vi "Run.vi"(8 "error in (no error)":errorcluster caption="entrée d'erreur (pas d'erreur)", 9 "labels_pred":string[][](array[string]), 10 "labels_true":string[][](array[string]), 11 "Contingency_Matrix.lvclass":refnum<class "Contingency_Matrix.lvclass">) -> (0 "error out":errorcluster caption="sortie d'erreur", 2 "Data":T1, 3 "Contingency_Matrix.lvclass":refnum<class "Contingency_Matrix.lvclass">)   [LabVIEW 2020, in "Contingency_Matrix.lvclass"]
doc: "Returns :\n\n- contingency : {array-like, sparse}, shape=[n_classes_true, n_classes_pred]\nMatrix such that is the number of samples in true class and in predicted class . If eps is None, the dtype of this array will be integer. If eps is given, the dtype will be float. Will be a scipy.sparse.csr_matrix if sparse=True."
uses:
  Contingency_Matrix.lvclass
  Contingency_Matrix.lvclass/Contingency_Matrix.ctl
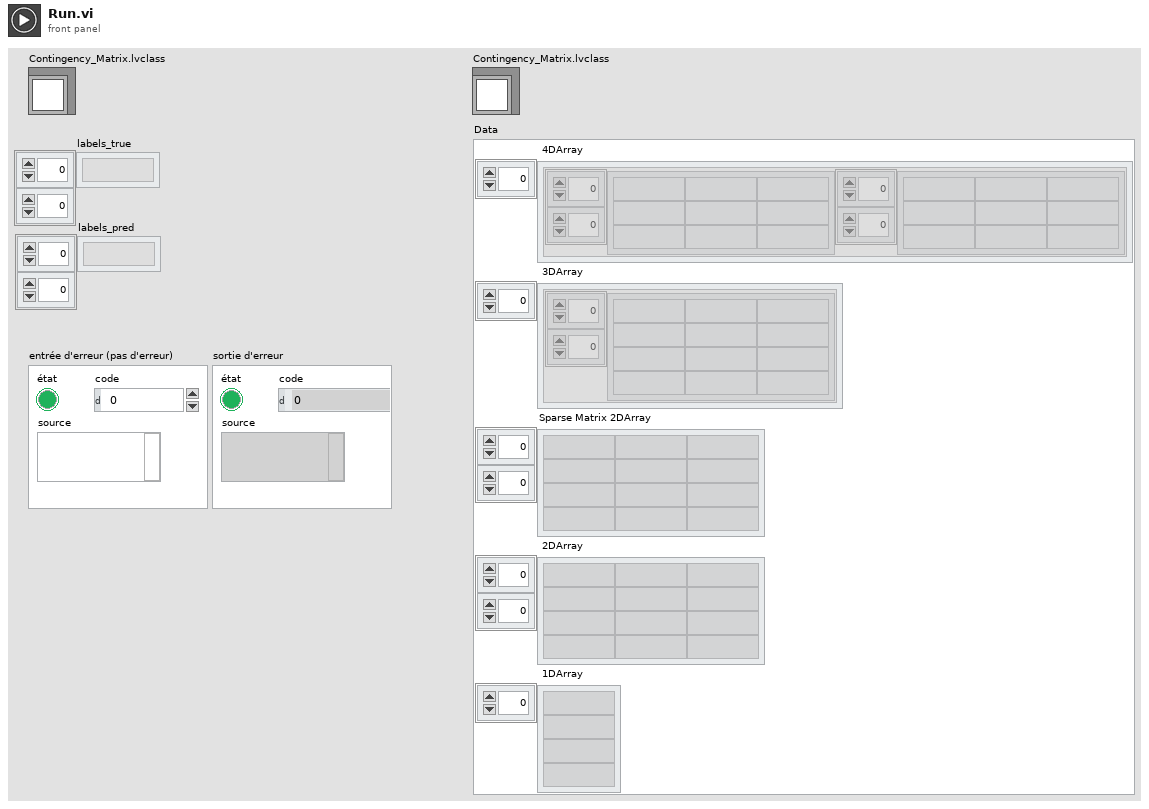
[diagram p1: front panel]
types:
  T1 = cluster{" 4DArray":cluster{"1":string[][], "2":string[][]}[], " 3DArray":cluster{"Tableau":string[][]}[], "Sparse Matrix 2DArray":string[][], " 2DArray":string[][], " 1DArray":string[]}
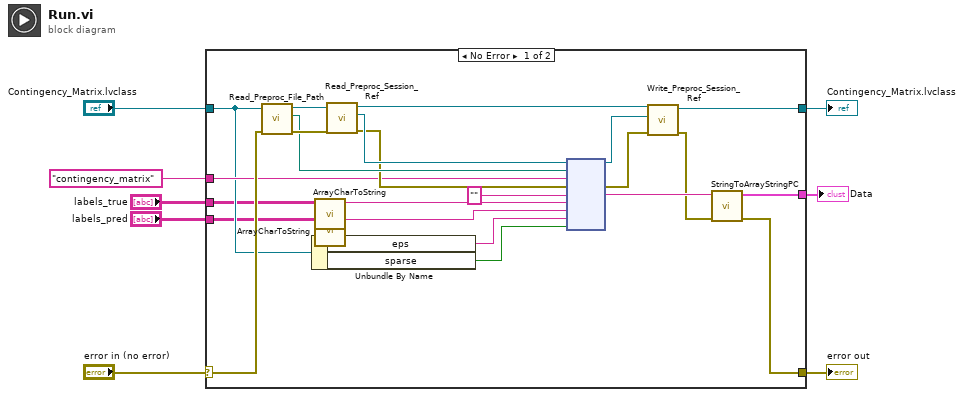
[diagram p0: block diagram]
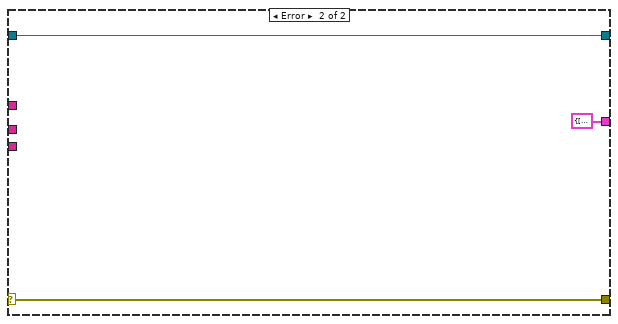
[diagram p2: hidden frame]
diagram:
  n1 = case shown="No Error" "error in (no error)" {
    selector: "error in (no error)" -> [w22 w34]
    tunnel: [w10 w34] -> w7
    tunnel: [w13 w33] -> w5
    tunnel: "Contingency_Matrix.lvclass" -> [w20 w33]
    tunnel: "contingency_matrix" -> [w21 _]
    tunnel: "labels_true" -> [w17 _]
    tunnel: "labels_pred" -> [w16 _]
    tunnel: [w9 T1 {" 4DArray"=[], " 3DArray"=[], "Sparse Matrix 2DArray"=[], " 2DArray"=[], " 1DArray"=[]} ("Data")] -> w1
    frame No Error {
      n2 = call-dynamic "Read_Preproc_File_Path.vi"("error in (no error)"=w22, "Python in"=w20) -> ("error out"=w30:errorcluster, "File_Path"=w29:path, "Python out"=w31:refnum<class "Contingency_Matrix.lvclass">)  [unwired: 7 in]
      n3 = Unbundle By Name(w20) -> ("eps"=w19:string, "sparse"=w18:bool)
      n4 = call "ArrayCharToString.vi"("TAB"=w17) -> ("Instruction"=w15:string)  [unwired: 10 in]
      n5 = call "ArrayCharToString.vi"("TAB"=w16) -> ("Instruction"=w14:string)  [unwired: 10 in]
      n6 = call-dynamic "Read_Preproc_Session_Ref.vi"("error in (no error)"=w30, "Python in"=w31) -> ("error out"=w27:errorcluster, "Session_ref"=w28:refnum<k35>, "Python out"=w26:refnum<class "Contingency_Matrix.lvclass">)  [unwired: 7 in]
      n7 = node(w28, w29, w21, w27, "", w15, w14, w19, w18) -> (w24:refnum<k35>, w25:errorcluster, w12:string)  [unwired: 4 in, 2 out]
      n8 = call-dynamic "Write_Preproc_Session_Ref.vi"("error in (no error)"=w25, "Session_ref"=w24, "Python in"=w26) -> ("error out"=w11:errorcluster, "Python out"=w13:refnum<class "Contingency_Matrix.lvclass">)  [unwired: 7 in]
      n9 = call "StringToArrayStringPC.vi"("sortie d'erreur"=w11, "Return value"=w12) -> ("sortie d'erreur"=w10:errorcluster, "Data"=w9:T1)  [unwired: 8 in]
    }
    frame Error {
    }
  }
  "error out" <- w7
  "Contingency_Matrix.lvclass" <- w5
  "Data" <- w1
